vi "Panel.vi"(11 "SinglePlotPanel in":refnum<class "SinglePlotPanel.lvclass">) -> ()   [LabVIEW 2021, in "MultiBluePlot.lvlib" / "SinglePlotPanel.lvclass"]
uses:
  SinglePlotPanel.lvclass
  C:/Program Files/National Instruments/LabVIEW 2021/vi.lib/IlluminatedG/IG OOPanel/OOPanel/Panel/Panel.lvclass
  SinglePlotPanel.lvclass/SinglePlotPanel.ctl
  <userlib>/Blue Origin/BluePlot (Open Source)/Classes/BluePlotHandle/BluePlotHandle.lvclass
  <userlib>/Blue Origin/BluePlot (Open Source)/Classes/BluePlotHandle/Shutdown.vi
  <userlib>/Blue Origin/BluePlot (Open Source)/Classes/BluePlotHandle/UI Visible.vi
  <vilib>/IlluminatedG/IG OOPanel/OOPanel/Panel/Panel.lvclass
  <userlib>/Blue Origin/BluePlot (Open Source)/BluePlot.lvlib
  C:/Code/open source/BluePlotMulti/Source/Classes/SinglePlotPanel/SinglePlotPanel.lvclass
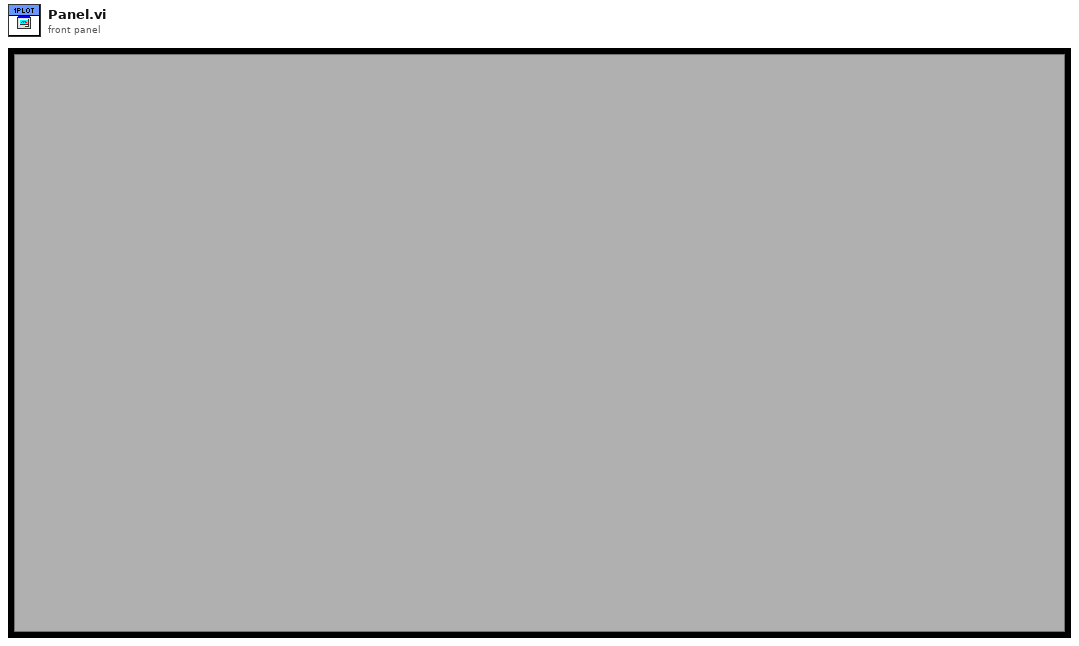
[diagram p1: front panel]
types:
  T1 = typedef "OOPanel.lvlib/Visibility State.ctl" = enum16{"Idle", "Closed", "Hidden", "Visible", "Subpanel", "Hidden Subpanel"}
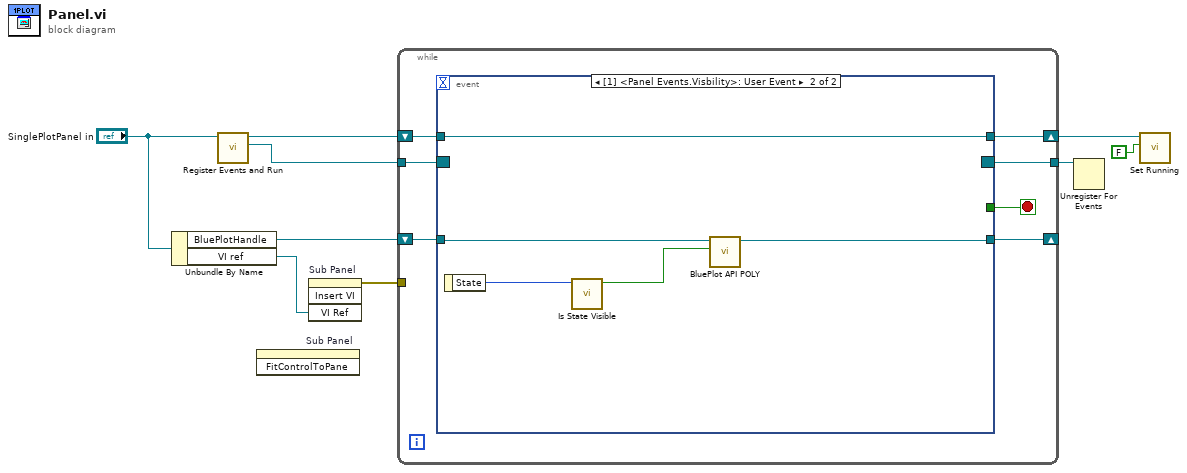
[diagram p0: block diagram]
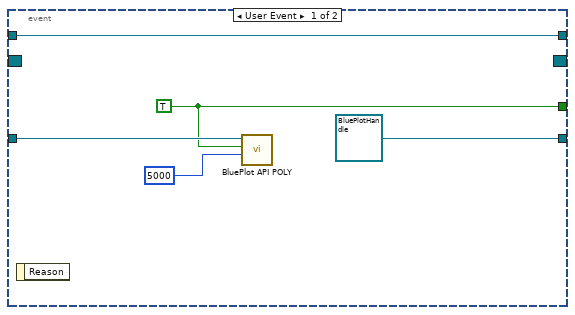
[diagram p2: hidden frame]
diagram:
  n1 = Unbundle By Name("SinglePlotPanel in") -> ("BluePlotHandle"=w2:refnum<class "BluePlotHandle.lvclass">, "VI ref"=w1:refnum<vi>)
  n2 = call <vilib>:"Register Events and Run.vi"("Panel in"="SinglePlotPanel in") -> ("Panel Event Reg"=w4:refnum<event-registration>, "Panel out"=w5:refnum<class "SinglePlotPanel.lvclass">)  [unwired: 8 in, 1 out]
  n3 = invoke on="Sub Panel" class="SubPnl" method="FitControlToPane"() -> ()  [unwired: 3 in, 3 out]
  n4 = invoke on="Sub Panel" class="SubPnl" method="Insert VI"("VI Ref"=w1) -> (error out=w7:errorcluster)  [unwired: 3 in, 3 out]
  n5 = while {
    shift-right: [w12] -> _
    shift-left: w2 -> [w13]
    tunnel: w7 -> [_]
    tunnel: w4 -> [w11]
    tunnel: [w10] -> w3
    shift-right: [w14] -> w9
    shift-left: w5 -> [w15]
    stop <- w16 stop-if-true
    n6 = event shown="[1] <Panel Events.Visbility>: User Event" {
      selector: w11 -> [_ _]
      dyn-events: [_ _] -> w10
      timeout: _ -> [_ _]
      tunnel: [w19 _] -> w16
      tunnel: w15 -> [w21 w22]
      tunnel: [w21 w22] -> w14
      tunnel: w13 -> [w20 w25]
      tunnel: [refnum<class "BluePlotHandle.lvclass"> refnum ("BluePlotHandle out") w24] -> w12
      event User Event {
        w19 = TRUE
        n7 = event-data() -> ()  [unwired: 1 in, 1 out]
        n8 = call-poly <userlib>:"BluePlot API POLY.vi"("wait timeout in ms (-1)"=5000, "Wait until shutdown? (F)"=w19, "BluePlotHandle in"=w20) -> ()  [unwired: 8 in, 1 out]
      }
      event User Event {
        n9 = event-data() -> ("State"=w23:T1)  [unwired: 1 in]
        n10 = call <vilib>:"Is State Visible.vi"("Visibility"=w23) -> ("Visible"=w26:bool)  [unwired: 10 in]
        n11 = call-poly <userlib>:"BluePlot API POLY.vi"("UI visible?"=w26, "BluePlotHandle in"=w25) -> ("BluePlotHandle out"=w24:refnum<class "BluePlotHandle.lvclass">)  [unwired: 8 in, 1 out]
      }
    }
  }
  n12 = Unregister For Events(event registration refnum=w3) -> ()  [unwired: 1 in, 1 out]
  n13 = call <vilib>:"Set Running.vi"("Running"=FALSE, "Panel in"=w9) -> ()  [unwired: 8 in, 2 out]
